vi "Rename and Replace Module VI.vi"(8 "error in (no error)":errorcluster, 10 "New Module/Lib Name":string, 11 "ProjectItem In":refnum<vi>) -> (0 "error out":errorcluster, 1 "Main VI Path":path, 2 "Main VI Name":string, 3 "ProjectItem Out":refnum<vi>)   [LabVIEW 2015, in "Generic Module Library.lvlib"]
uses:
  Generic Module Library.lvlib
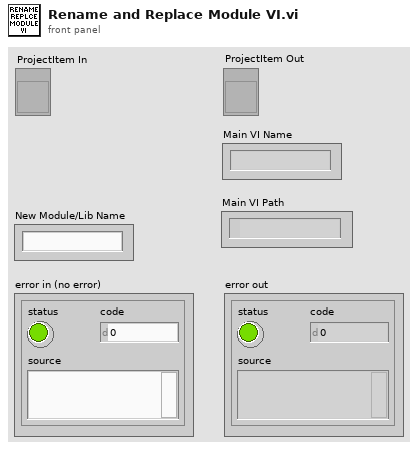
[diagram p1: front panel]
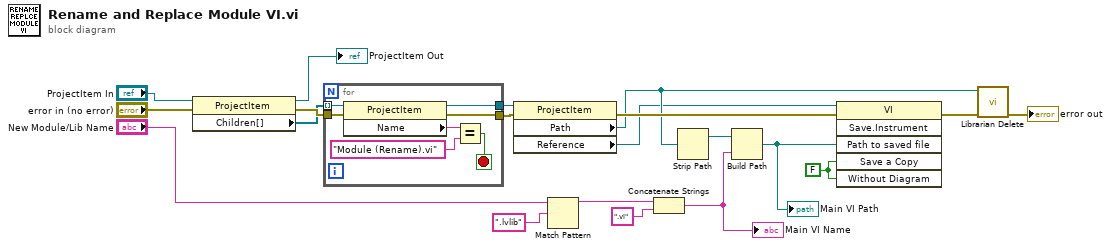
[diagram p0: block diagram]
diagram:
  w7 = FALSE ("Save a Copy")
  n1 = property on="Property Node" class="ProjectItem"(reference="ProjectItem In", error in="error in (no error)") -> (reference out=→"ProjectItem Out":refnum<vi>, error out=w20:errorcluster, "Children[]"=w5:refnum<vi>[])
  n2 = for {
    tunnel: w5 -> [w27] mode=indexing
    tunnel: [w23] -> w6
    tunnel: [w22] -> w19
    tunnel: w20 -> [w21]
    stop <- w24 stop-if-true
    n3 = property class="ProjectItem"(reference=w27, error in=w21) -> (reference out=w23:refnum<vi>, error out=w22:errorcluster, "Name"=w26:string)
    n4 = Equal?(x=w26, y="Module (Rename).vi") -> (x = y?=w24:bool)
  }
  n5 = property class="ProjectItem"(reference=w6, error in=w19) -> (error out=w18:errorcluster, "Path"=w9:path, "Reference"=w8:refnum<vi>)  [unwired: 1 out]
  n6 = Match Pattern(string="New Module/Lib Name", regular expression=".lvlib") -> (before substring=w15:string)  [unwired: 1 in, 3 out]
  n7 = Concatenate Strings(w15, ".vi" ("string")) -> (w11:string)
  "Main VI Name" <- w11
  n8 = Strip Path(path=w9) -> (stripped path=w10:path)  [unwired: 1 out]
  n9 = Build Path(base path=w10, name or relative path=w11) -> (appended path=w13:path)
  "Main VI Path" <- w13
  n10 = invoke class="VI" method="Save.Instrument"(reference=w8, error in=w18, "Path to saved file"=w13, "Save a Copy"=w7, "Without Diagram"=w7) -> (error out=w2:errorcluster)  [unwired: 1 in, 5 out]
  n11 = call <vilib>:"Librarian Delete.vi"("error in (no error)"=w2, "path"=w9) -> ("error out"=→"error out":errorcluster)  [unwired: 9 in]
